vi "Compile Datalog Array sub_VI.vi"(2 "XY Cluster":T1={"X Data"={"Complete?"=FALSE, "Motor Params"={"Duty %"=0.0, "X Freq"=0.0, "FWD/RVS"=FALSE}, "SP"={"Accel"=0.0, "Decel"=0.0, "Speed"=0.0}, "State"=enum."Stop", "Input"={"Coord"=0.0, "Tol"=0.0, "Accel"=0.0, "Decel"=0.0, "Max Speed"=0.0}, "Path"={"V plan"=[], "V actual"=[], "S actual"=[], "a actual"=[], "Profile"=enum."Triangular", "Decel Dist"=0.0, "Accel Dist"=0.0, "Cruise V"=0.0, "Cruise Dist"=0.0}, "PID"={"Kc"=0.0, "Ti"=0.0, "Td"=0.0}, "Motion"={"Speed"=0.0, "Dist"=0.0, "Acceleration"=0.0, "Dist to target"=0.0}}, "Y Data"={"Complete?"=FALSE, "Motor Params"={"Duty %"=0.0, "Freq"=0.0, "FWD/RVS"=FALSE}, "SP"={"Y Accel"=0.0, "Y Decel"=0.0, "Speed"=0.0}, "State"=enum."Stop", "Input"={"Coord"=0.0, "Tol"=0.0, "Accel"=0.0, "Decel"=0.0, "Max Speed"=0.0}, "Path"={"V plan"=[], "V actual"=[], "S actual"=[], "a actual"=[], " Profile"=enum."Triangular", "Decel Dist"=0.0, "Accel Dist"=0.0, "Cruise V"=0.0, "Cruise Dist"=0.0}, "PID"={"Kc"=0.0, "Ti"=0.0, "Td"=0.0}, "Motion"={"Speed"=0.0, "Dist"=0.0, "Acceleration"=0.0, "Dist to target"=0.0}}, "Timing"={"Runtime"=0.0, "Loop time"=0.0, "Loop iter"=0, "Tick"=0.0}, "stop"=FALSE} {"Y Data"."Input"."Tol" min=0.0; "X Data"."Input"."Tol" min=0.0}, 3 "Initialised Array":dbl[][](array[numeric])) -> (0 "Data Array":dbl[][](array[numeric]))   [LabVIEW 2017]
uses:
  XY Cluster.ctl
  Motor Status Enum.ctl
  Motion Type Def.ctl
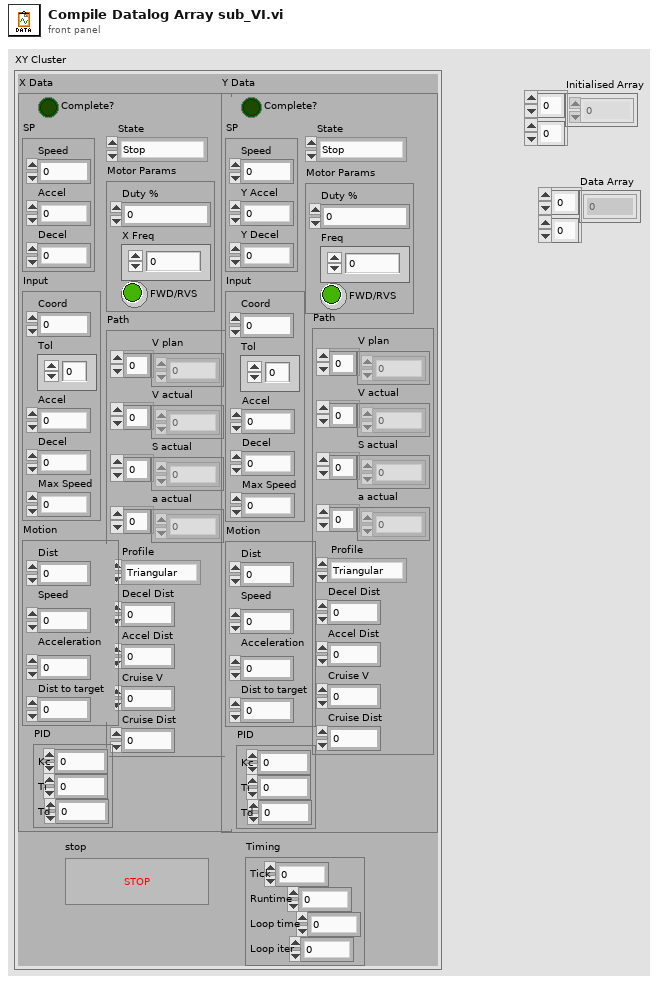
[diagram p1: front panel]
types:
  T1 = typedef "XY Cluster.ctl" = cluster{"X Data":cluster{"Complete?":bool, "Motor Params":cluster{"Duty %":dbl, "X Freq":dbl, "FWD/RVS":bool}, "SP":cluster{"Accel":dbl, "Decel":dbl, "Speed":dbl}, "State":T2, "Input":cluster{"Coord":dbl, "Tol":dbl, "Accel":dbl, "Decel":dbl, "Max Speed":dbl}, "Path":cluster{"V plan":dbl[], "V actual":dbl[], "S actual":dbl[], "a actual":dbl[], "Profile":T3, "Decel Dist":dbl, "Accel Dist":dbl, "Cruise V":dbl, "Cruise Dist":dbl}, "PID":cluster{"Kc":dbl, "Ti":dbl, "Td":dbl}, "Motion":cluster{"Speed":dbl, "Dist":dbl, "Acceleration":dbl, "Dist to target":dbl}}, "Y Data":cluster{"Complete?":bool, "Motor Params":cluster{"Duty %":dbl, "Freq":dbl, "FWD/RVS":bool}, "SP":cluster{"Y Accel":dbl, "Y Decel":dbl, "Speed":dbl}, "State":T2, "Input":cluster{"Coord":dbl, "Tol":dbl, "Accel":dbl, "Decel":dbl, "Max Speed":dbl}, "Path":cluster{"V plan":dbl[], "V actual":dbl[], "S actual":dbl[], "a actual":dbl[], " Profile":T3, "Decel Dist":dbl, "Accel Dist":dbl, "Cruise V":dbl, "Cruise Dist":dbl}, "PID":cluster{"Kc":dbl, "Ti":dbl, "Td":dbl}, "Motion":cluster{"Speed":dbl, "Dist":dbl, "Acceleration":dbl, "Dist to target":dbl}}, "Timing":cluster{"Runtime":dbl, "Loop time":dbl, "Loop iter":i32, "Tick":dbl}, "stop":bool}
  T2 = typedef "Motor Status Enum.ctl" = enum16{"Update I/O", "Stop", "Steady Speed", "Accelerate", "Decelerate", "Drive Motor"}
  T3 = typedef "Motion Type Def.ctl" = enum16{"Trapezodial", "Triangular"}
  T4 = cluster{"Complete?":bool, "Motor Params":cluster{"Duty %":dbl, "X Freq":dbl, "FWD/RVS":bool}, "SP":cluster{"Accel":dbl, "Decel":dbl, "Speed":dbl}, "State":T2, "Input":cluster{"Coord":dbl, "Tol":dbl, "Accel":dbl, "Decel":dbl, "Max Speed":dbl}, "Path":cluster{"V plan":dbl[], "V actual":dbl[], "S actual":dbl[], "a actual":dbl[], "Profile":T3, "Decel Dist":dbl, "Accel Dist":dbl, "Cruise V":dbl, "Cruise Dist":dbl}, "PID":cluster{"Kc":dbl, "Ti":dbl, "Td":dbl}, "Motion":cluster{"Speed":dbl, "Dist":dbl, "Acceleration":dbl, "Dist to target":dbl}}
  T5 = cluster{"Complete?":bool, "Motor Params":cluster{"Duty %":dbl, "Freq":dbl, "FWD/RVS":bool}, "SP":cluster{"Y Accel":dbl, "Y Decel":dbl, "Speed":dbl}, "State":T2, "Input":cluster{"Coord":dbl, "Tol":dbl, "Accel":dbl, "Decel":dbl, "Max Speed":dbl}, "Path":cluster{"V plan":dbl[], "V actual":dbl[], "S actual":dbl[], "a actual":dbl[], " Profile":T3, "Decel Dist":dbl, "Accel Dist":dbl, "Cruise V":dbl, "Cruise Dist":dbl}, "PID":cluster{"Kc":dbl, "Ti":dbl, "Td":dbl}, "Motion":cluster{"Speed":dbl, "Dist":dbl, "Acceleration":dbl, "Dist to target":dbl}}
  T6 = cluster{"Runtime":dbl, "Loop time":dbl, "Dist":dbl, "Duty %":dbl, "X Freq":dbl, "Dist":dbl, "Freq":dbl, "Accel":dbl, "Decel":dbl, "Accel":dbl, "Decel":dbl, "Coord":dbl, "Coord":dbl, "Velocity (mm/s)":dbl, "Acceleration (mm/s^2)":dbl, "Velocity (mm/s)":dbl, "Acceleration (mm/s^2)":dbl}
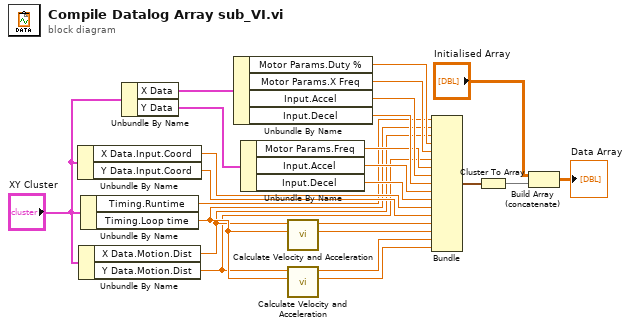
[diagram p0: block diagram]
diagram:
  n1 = Unbundle By Name("XY Cluster") -> ("X Data.Input.Coord"=w7:dbl, "Y Data.Input.Coord"=w6:dbl)
  n2 = Unbundle By Name("XY Cluster") -> ("X Data.Motion.Dist"=w2:dbl, "Y Data.Motion.Dist"=w1:dbl)
  n3 = Unbundle By Name("XY Cluster") -> ("Timing.Runtime"=w5:dbl, "Timing.Loop time"=w4:dbl)
  n4 = Unbundle By Name("XY Cluster") -> ("X Data"=w12:T4, "Y Data"=w11:T5)
  n5 = Unbundle By Name(w12) -> ("Motor Params.Duty %"=w16:dbl, "Motor Params.X Freq"=w15:dbl, "Input.Accel"=w14:dbl, "Input.Decel"=w13:dbl)
  n6 = Unbundle By Name(w11) -> ("Motor Params.Freq"=w10:dbl, "Input.Accel"=w9:dbl, "Input.Decel"=w8:dbl)
  n7 = call "Calculate Velocity and Acceleration.vi"("Loop Runtime (s)"=w4, "Displacement (mm)"=w2) -> ("Acceleration (mm/s^2)"=w21:dbl, "Velocity (mm/s)"=w20:dbl)  [unwired: 8 in]
  n8 = call "Calculate Velocity and Acceleration.vi"("Loop Runtime (s)"=w4, "Displacement (mm)"=w1) -> ("Acceleration (mm/s^2)"=w23:dbl, "Velocity (mm/s)"=w22:dbl)  [unwired: 8 in]
  n9 = Bundle("Runtime"=w5, "Loop time"=w4, "Dist"=w2, "Duty %"=w16, "X Freq"=w15, "Dist"=w1, "Freq"=w10, "Accel"=w14, "Decel"=w13, "Accel"=w9, "Decel"=w8, "Coord"=w7, "Coord"=w6, "Velocity (mm/s)"=w20, "Acceleration (mm/s^2)"=w21, "Velocity (mm/s)"=w22, "Acceleration (mm/s^2)"=w23) -> (w18:T6)  [unwired: 1 in]
  n10 = Cluster To Array(cluster=w18) -> (array=w17:dbl[])
  n11 = Build Array (concatenate)("Initialised Array", w17) -> (→"Data Array":dbl[][])
